vi "stopCI2_img.vi"   [LabVIEW 2013]
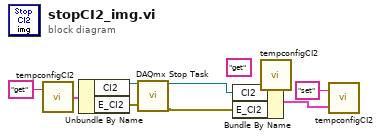
[diagram p0: block diagram]
diagram:
  (unwired) "get" ("command")
  n1 = call "tempconfigCI2.vi"("command"="get") -> ("Temp Config out"=w8:cluster{"CI2":refnum<k21>, "E_CI2":errorcluster})  [unwired: 1 in]
  n2 = Unbundle By Name(w8) -> ("CI2"=w7:refnum<k21>, "E_CI2"=w6:errorcluster)
  n3 = call <vilib>:"DAQmx Stop Task.vi"("task/channels in"=w7, "error in"=w6) -> ("task out"=w2:refnum<k21>, "error out"=w1:errorcluster)  [unwired: 12 in]
  n4 = call "tempconfigCI2.vi"() -> ("Temp Config out"=w4:cluster{"CI2":refnum<k21>, "E_CI2":errorcluster})  [unwired: 2 in]
  n5 = Bundle By Name(cluster=w4, "CI2"=w2, "E_CI2"=w1) -> (w3:cluster{"CI2":refnum<k21>, "E_CI2":errorcluster})
  n6 = call "tempconfigCI2.vi"("Temp Config in"=w3, "command"="set") -> ()  [unwired: 1 out]
